vi "User Event Print.vi"(7 "Options":T1(ring), 8 "error in (no error)":errorcluster, 9 "add EOL?":bool, 11 "String to Print":string) -> (0 "error out":errorcluster, 3 "Print":refnum<user-event>)   [LabVIEW 2017]
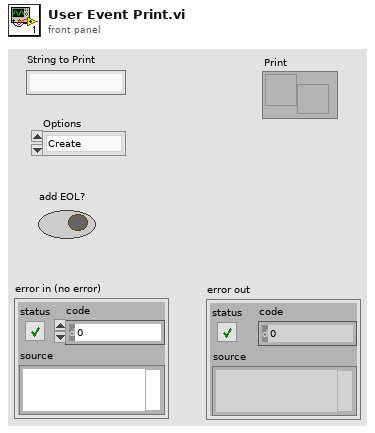
[diagram p1: front panel]
types:
  T1 = enum16{"Create", "Get Reference", "Print", "Close"}
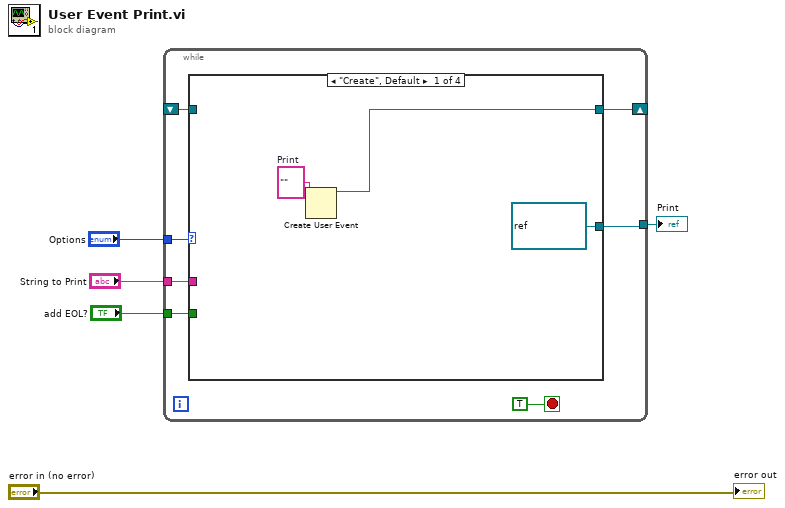
[diagram p0: block diagram]
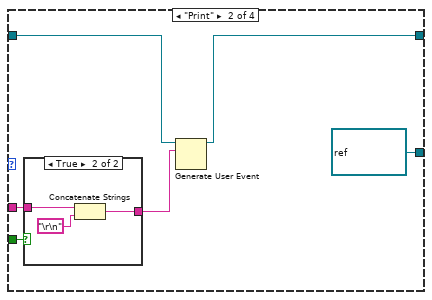
[diagram p2: hidden frame]
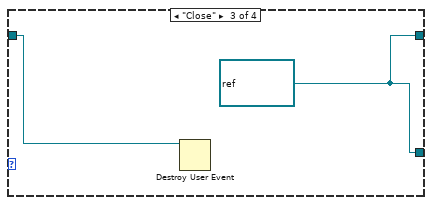
[diagram p4: hidden frame]
diagram:
  n1 = while {
    tunnel: "Options" -> [w11]
    tunnel: "String to Print" -> [w10]
    tunnel: "add EOL?" -> [w9]
    shift-right: [w8] -> _
    shift-left: _ -> [w7]
    tunnel: [w6] -> w1
    stop <- TRUE stop-if-true
    n2 = case shown="\"Create\", Default" w11 {
      tunnel: w10 -> [_ w21 _ _]
      tunnel: w9 -> [_ w19 _ _]
      tunnel: [w14 w17 w26 w28] -> w8
      tunnel: w7 -> [_ w18 w27 w28]
      tunnel: [refnum<user-event> refnum ("Print") refnum<user-event> refnum ("Print") w26 w28] -> w6
      frame "Create", Default {
        w15 = ""  # Print
        n3 = Create User Event(user event datatype=w15) -> (user event=w14:refnum<user-event>)  [unwired: 1 in, 1 out]
      }
      frame "Print" {
        n4 = case shown="True" w19 {
          tunnel: w21 -> [w22 w25]
          tunnel: [w22 w24] -> w20
          frame False {
          }
          frame True {
            n5 = Concatenate Strings(w25, "\r\n") -> (w24:string)
          }
        }
        n6 = Generate User Event(user event=w18, event data cluster=w20) -> (user event out=w17:refnum<user-event>)  [unwired: 2 in, 1 out]
      }
      frame "Close" {
        w26 = refnum<user-event> refnum ("Print")
        n7 = Destroy User Event(user event=w27) -> ()  [unwired: 1 in, 1 out]
      }
      frame "Get Reference" {
      }
    }
  }
  "Print" <- w1
  "error out" <- "error in (no error)"
